vi "Build.vi"(8 "error in (no error)":errorcluster, 11 "CD Build Tools in":refnum<class "Project Build Tools.lvclass">) -> (0 "error out":errorcluster, 2 "Generated files":path[][](array[path]), 3 "CD Build Tools out":refnum<class "Project Build Tools.lvclass">)   [LabVIEW 2019, in "Project Build Tools.lvclass"]
uses:
  Project Build Tools.lvclass
  Project Build Tools.lvclass/Project Build Tools.ctl
  <vilib>/AppBuilder/AB_API_Simple/Build (path).vi
  <vilib>/AppBuilder/AB_API_Simple/NI_App_Builder_API.lvlib
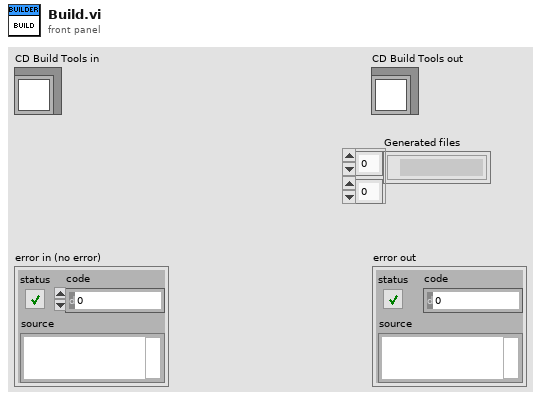
[diagram p1: front panel]
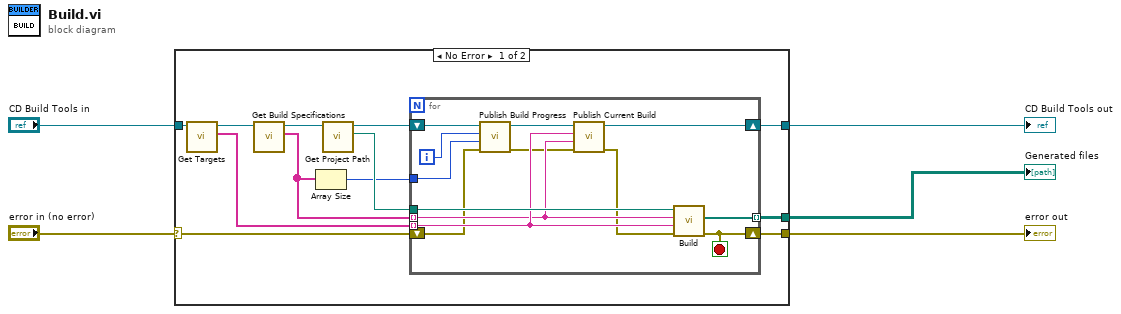
[diagram p0: block diagram]
diagram:
  n1 = case shown="No Error" "error in (no error)" {
    selector: "error in (no error)" -> [w11 w31]
    tunnel: [w7 w32] -> w2
    tunnel: [w15 w31] -> w3
    tunnel: "CD Build Tools in" -> [w14 w32]
    tunnel: [w6 _] -> w1
    frame No Error {
      n2 = call "Get Targets.vi"("CD Build Tools in"=w14) -> ("Targets"=w12:string[], "CD Build Tools out"=w13:refnum<class "Project Build Tools.lvclass">)  [unwired: 9 in]
      n3 = call "Get Build Specifications.vi"("CD Build Tools in"=w13) -> ("Build Specifications"=w10:string[], "CD Build Tools out"=w16:refnum<class "Project Build Tools.lvclass">)  [unwired: 9 in]
      n4 = Array Size(array=w10) -> (size(s)=w9:i32)
      n5 = call "Get Project Path.vi"("CD Build Tools in"=w16) -> ("Project Path"=w17:path, "CD Build Tools out"=w8:refnum<class "Project Build Tools.lvclass">)  [unwired: 9 in]
      n6 = for {
        tunnel: w17 -> [w30]
        shift-right: [w29] -> w15
        shift-left: w11 -> [w23]
        tunnel: w10 -> [w27] mode=indexing
        tunnel: w12 -> [w28] mode=indexing
        tunnel: w9 -> [w24]
        shift-right: [w20] -> w7
        shift-left: w8 -> [w26]
        tunnel: [w18] -> w6 mode=indexing
        i -> [w25]
        stop <- w29 stop-if-true
        n7 = call "Publish Build Progress.vi"("error in (no error)"=w23, "Total Number of Builds"=w24, "Current Iteration"=w25, "CD Build Tools in"=w26) -> ("error out"=w21:errorcluster, "CD Build Tools out"=w22:refnum<class "Project Build Tools.lvclass">)  [unwired: 6 in]
        n8 = call "Publish Current Build.vi"("error in (no error)"=w21, "Build Specification Name"=w27, "Target"=w28, "CD Build Tools in"=w22) -> ("error out"=w19:errorcluster, "CD Build Tools out"=w20:refnum<class "Project Build Tools.lvclass">)  [unwired: 6 in]
        n9 = call-poly <vilib>:"Build.vi"("error in (no error)"=w19, "Name of target (My Computer)"=w28, "Name of build specification (if empty: build all)"=w27, "Path to project"=w30) -> ("error out"=w29:errorcluster, "Generated files"=w18:path[])  [unwired: 6 in]
      }
    }
    frame Error {
    }
  }
  "error out" <- w3
  "CD Build Tools out" <- w2
  "Generated files" <- w1
